vi "exercice7-1.vi"() -> ()   [LabVIEW 2013]
panel:
  in  "Numérique":dbl
  in  "Chaîne":string
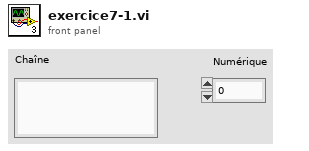
[diagram p1: front panel]
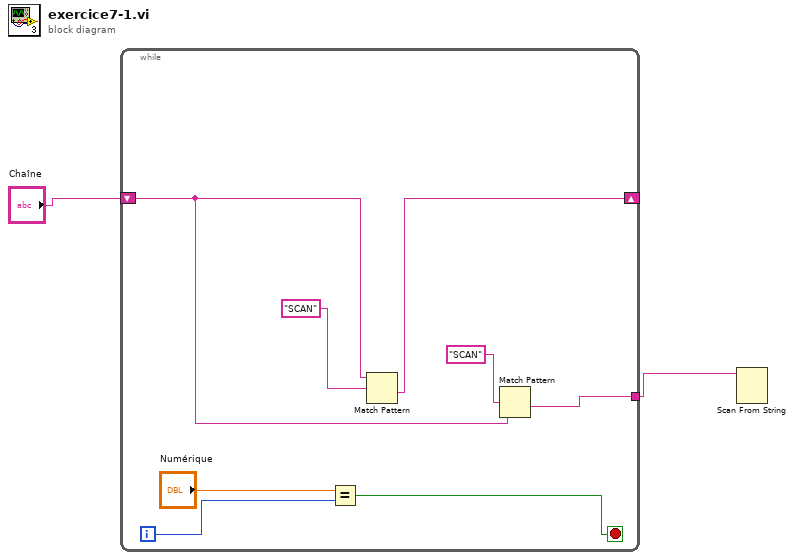
[diagram p0: block diagram]
diagram:
  n1 = while {
    shift-right: [w6] -> _
    shift-left: "Chaîne" -> [w4]
    tunnel: [w3] -> w1
    i -> [w9]
    stop <- w7 stop-if-true
    n2 = Equal?(x="Numérique", y=w9) -> (x = y?=w7:bool)
    n3 = Match Pattern(string=w4, regular expression="SCAN") -> (after substring=w6:string)  [unwired: 1 in, 3 out]
    n4 = Match Pattern(string=w4, regular expression="SCAN") -> (after substring=w3:string)  [unwired: 1 in, 3 out]
  }
  n5 = Scan From String(input string=w1) -> ()  [unwired: 5 in, 3 out]
